vi "Set Main Ctl Ref and VI Ref.vi"(8 "error in (no error)":errorcluster, 10 "Main Ctl and VI Ref":T1, 11 "ScriptSetting in":refnum<class "ScriptSetting.lvclass">) -> (0 "error out":errorcluster, 3 "ScriptSetting out":refnum<class "ScriptSetting.lvclass">)   [LabVIEW 2015, in "ScriptSetting.lvclass"]
uses:
  ScriptSetting.lvclass
  Type Definitions/Main Controls and VI Ref in ScriptsConfiguration.ctl
  ScriptSetting.lvclass/ScriptSetting.ctl
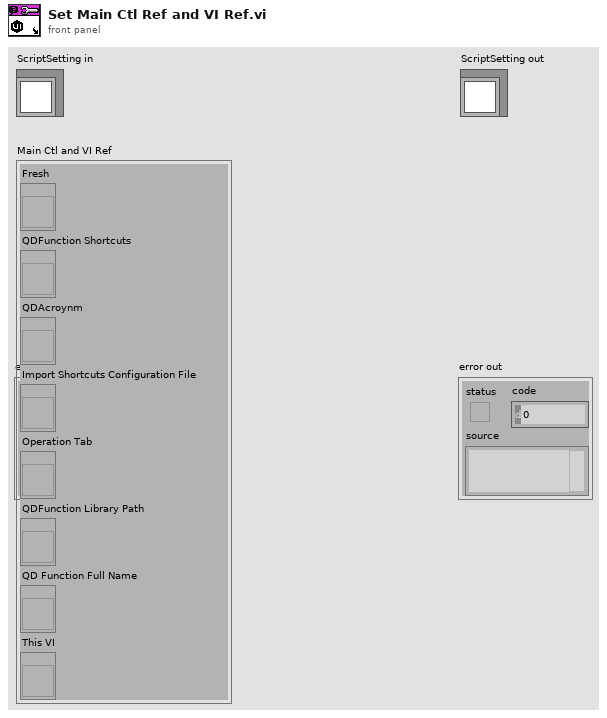
[diagram p1: front panel]
types:
  T1 = typedef "ScriptSetting.lvclass/Main Controls and VI Ref in ScriptsConfiguration.ctl" = cluster{"Fresh":refnum<vi>, "QDFunction Shortcuts":refnum<vi>, "QDAcroynm":refnum<vi>, "Import Shortcuts Configuration File":refnum<vi>, "Operation Tab":refnum<vi>, "QDFunction Library Path":refnum<vi>, "QD Function Full Name":refnum<vi>, "This VI":refnum<vi>}
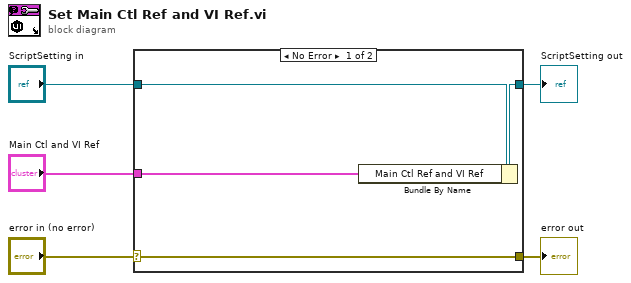
[diagram p0: block diagram]
diagram:
  n1 = case shown="No Error" "error in (no error)" {
    selector: "error in (no error)" -> [w9 w10]
    tunnel: [w9 w10] -> w4
    tunnel: [w7 w11] -> w2
    tunnel: "ScriptSetting in" -> [w8 w11]
    tunnel: "Main Ctl and VI Ref" -> [w6 _]
    frame No Error {
      n2 = Bundle By Name(cluster=w8, "Main Ctl Ref and VI Ref"=w6) -> (w7:refnum<class "ScriptSetting.lvclass">)
    }
    frame Error {
    }
  }
  "error out" <- w4
  "ScriptSetting out" <- w2
